vi "Write Delay Before Leaving.vi"(8 "error in (no error)":errorcluster, 10 "Delay Before Leaving [s]":dbl, 11 "Customer In":refnum<class "Customer.lvclass">) -> (0 "error out":errorcluster, 3 "Customer Out":refnum<class "Customer.lvclass">)   [LabVIEW 2020, in "Customer.lvclass"]
uses:
  Customer.lvclass
  Customer.lvclass/Customer.ctl
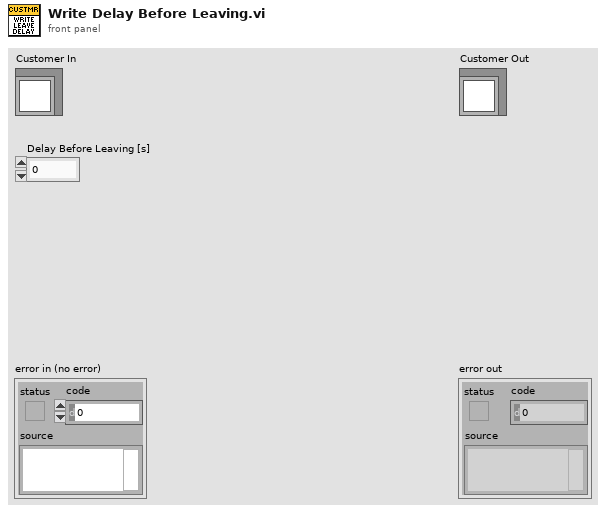
[diagram p1: front panel]
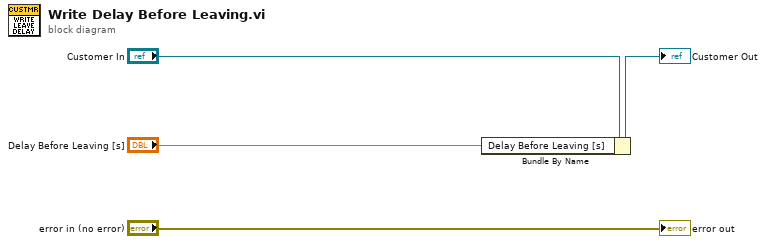
[diagram p0: block diagram]
diagram:
  n1 = Bundle By Name(cluster="Customer In", "Delay Before Leaving [s]"="Delay Before Leaving [s]") -> (→"Customer Out":refnum<class "Customer.lvclass">)
  "error out" <- "error in (no error)"
